vi "Settings Dialog.vi"(8 "error in (no error)":errorcluster, 11 "Settings in":T1={"Hardware Configuration"={"Sensor Channels"="", "Max Input"=10.0, "Min Input"=-10.0, "Sample Rate"=1000.0, "DAQmx Task"="", "Reference Channels"=""}, "Ga"=0.0, "Gv"=0.0, "ExportPath"=""}) -> (0 "error out":errorcluster, 1 "Cancelled?":bool=TRUE, 2 "UI Refresh Needed?":bool, 3 "Settings out":T1={"Hardware Configuration"={"Sensor Channels"="", "Max Input"=10.0, "Min Input"=-10.0, "Sample Rate"=1000.0, "DAQmx Task"="", "Reference Channels"=""}, "Ga"=0.0, "Gv"=0.0, "ExportPath"=""})   [LabVIEW 2017, in "Settings.lvlib"]
doc: "Dialog for selecting user specified settings."
uses:
  Settings.lvlib
  Settings.ctl
  Acquisition/Hardware Configuration.ctl
  <vilib>/Utility/xml.llb/Write to XML File(string).vi
  Acquisition/Acquisition.lvlib
panel:
  in  "Export Path":path
  in  "Reference G[V/m/s^2]":dbl=1000.0
  in  "Target G[V/m/s]":dbl=-10.0
  in  "Reference Channel":tag="Dev1/ai0"
  in  "Sample Rate":dbl=1000.0
  in  "Minimum Input":dbl=-10.0
  in  "Maximum Input":dbl=10.0
  in  "Sensor Channels":tag="Dev1/ai0"
  in  "Cancel Button":bool
  in  "OK Button":bool
  # "Non visible portion of dialog (needed for connector pane)."
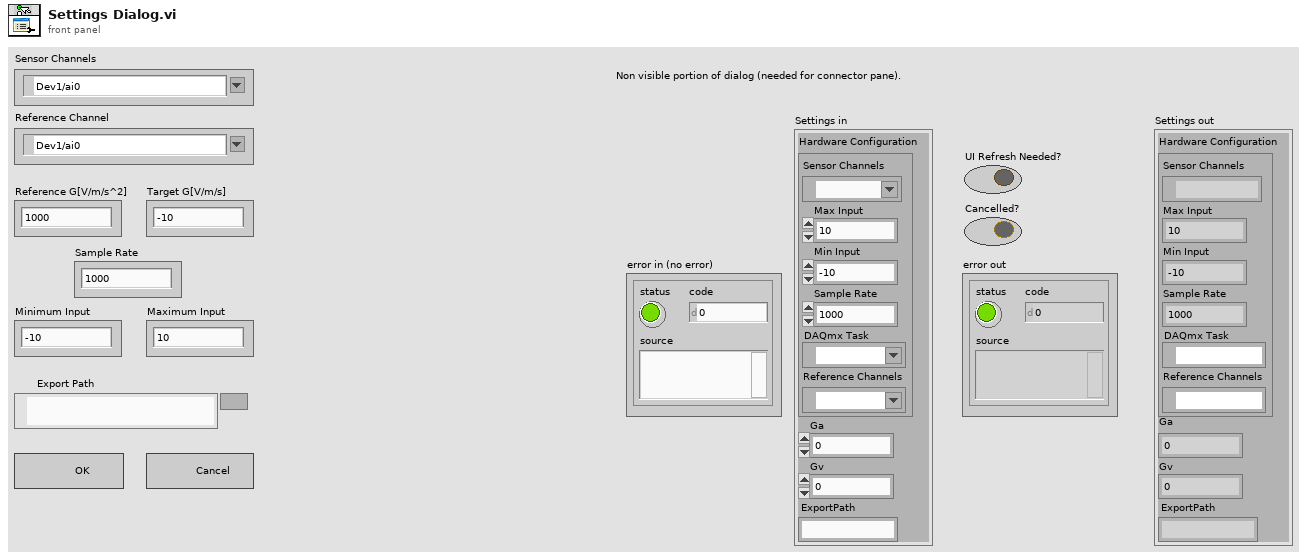
[diagram p1: front panel]
types:
  T1 = typedef "Settings.lvlib/Settings.ctl" = cluster{"Hardware Configuration":T2, "Ga":dbl, "Gv":dbl, "ExportPath":string}
  T2 = typedef "Acquisition.lvlib/Hardware Configuration.ctl" = cluster{"Sensor Channels":tag, "Max Input":dbl, "Min Input":dbl, "Sample Rate":dbl, "DAQmx Task":refnum<k21>, "Reference Channels":tag}
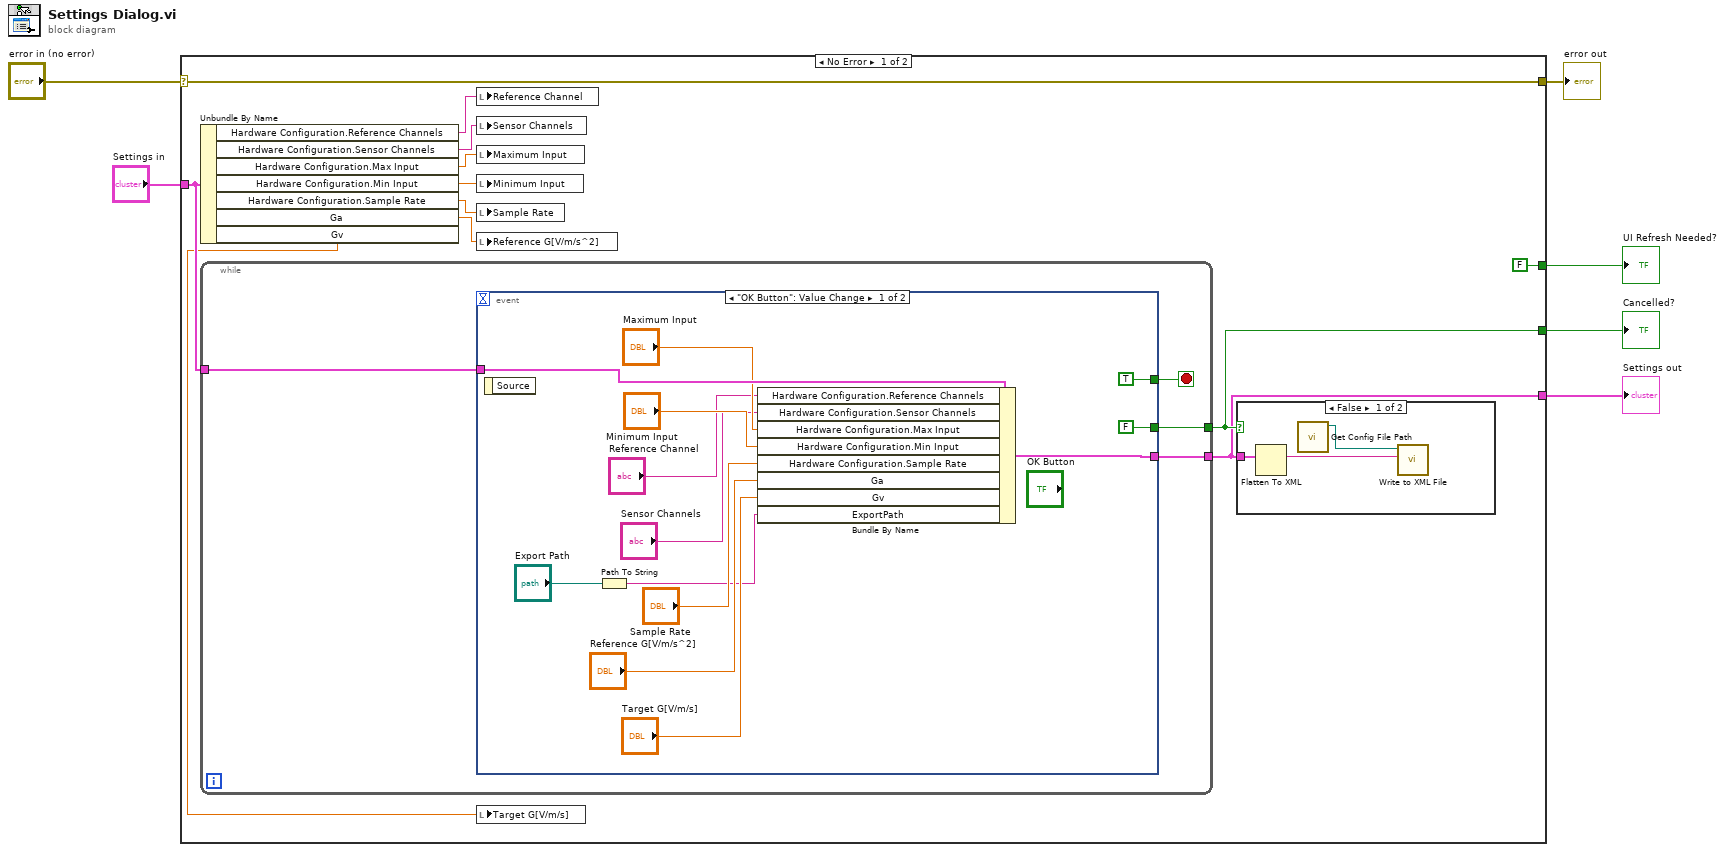
[diagram p0: block diagram]
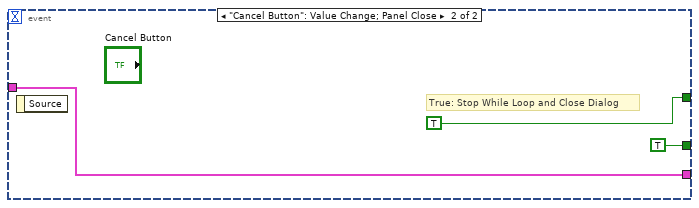
[diagram p2: hidden frame]
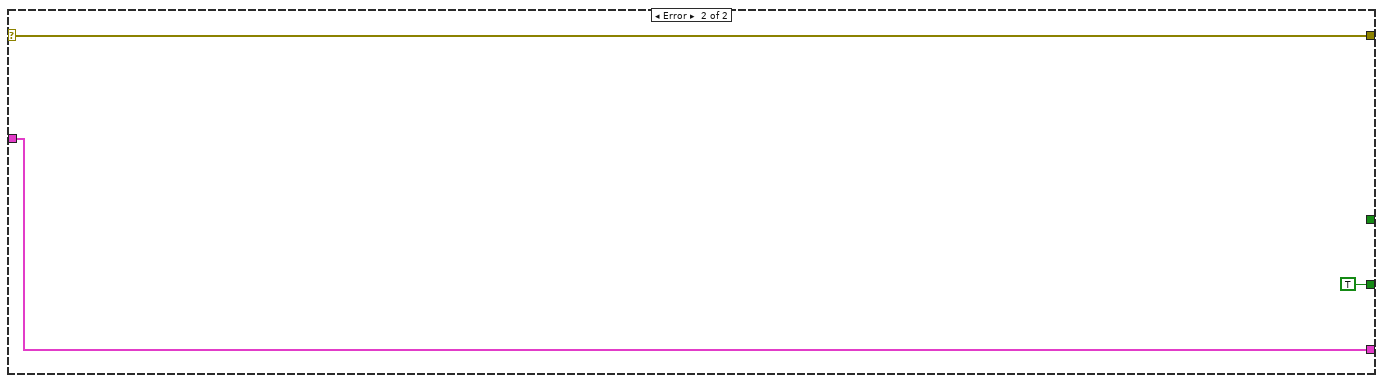
[diagram p4: hidden frame]
diagram:
  n1 = case shown="No Error" "error in (no error)" {
    selector: "error in (no error)" -> [w18 w44]
    tunnel: [w18 w44] -> w6
    tunnel: "Settings in" -> [w10 w43]
    tunnel: [w15 w43] -> w1
    tunnel: [FALSE ("UI Refresh Needed?") _] -> w4
    tunnel: [w16 TRUE ("UI Refresh Needed?")] -> w3
    frame No Error {
      n2 = Unbundle By Name(w10) -> ("Hardware Configuration.Reference Channels"=w9:tag, "Hardware Configuration.Sensor Channels"=w11:tag, "Hardware Configuration.Max Input"=w12:dbl, "Hardware Configuration.Min Input"=w13:dbl, "Hardware Configuration.Sample Rate"=w14:dbl, "Ga"=w8:dbl, "Gv"=w7:dbl)
      n3 = while {
        tunnel: [w22] -> w16
        tunnel: [w21] -> w15
        tunnel: w10 -> [w20]
        stop <- w19 stop-if-true
        n4 = event shown="[0] \"OK Button\": Value Change" {
          selector: _ -> [_ _]
          dyn-events: _ -> [_ _]
          timeout: _ -> [_ _]
          tunnel: [w33 w38] -> w21
          tunnel: w20 -> [w32 w38]
          tunnel: [FALSE ("UI Refresh Needed?") TRUE ("UI Refresh Needed?")] -> w22
          tunnel: [TRUE TRUE] -> w19
          event "OK Button": Value Change {
            n5 = event-data() -> ()  [unwired: 1 in, 1 out]
            n6 = Path To String(path="Export Path") -> (string=w23:string)
            n7 = Bundle By Name(cluster=w32, "Hardware Configuration.Reference Channels"="Reference Channel", "Hardware Configuration.Sensor Channels"="Sensor Channels", "Hardware Configuration.Max Input"="Maximum Input", "Hardware Configuration.Min Input"="Minimum Input", "Hardware Configuration.Sample Rate"="Sample Rate", "Ga"="Reference G[V/m/s^2]", "Gv"="Target G[V/m/s]", "ExportPath"=w23) -> (w33:T1)
          }
          event "Cancel Button": Value Change; Panel Close {
            # "True: Stop While Loop and Close Dialog"
            n8 = event-data() -> ()  [unwired: 1 in, 1 out]
          }
        }
      }
      n9 = local write "Reference Channel"(w9) -> ()
      n10 = local write "Sensor Channels"(w11) -> ()
      n11 = local write "Maximum Input"(w12) -> ()
      n12 = local write "Minimum Input"(w13) -> ()
      n13 = local write "Sample Rate"(w14) -> ()
      n14 = local write "Reference G[V/m/s^2]"(w8) -> ()
      n15 = local write "Target G[V/m/s]"(w7) -> ()
      n16 = case shown="False" w16 {
        tunnel: w15 -> [w40 _]
        frame False {
          n17 = Flatten To XML(anything=w40) -> (xml string=w39:string)
          n18 = call "Get Config File Path.vi"() -> ("XML File Path"=w41:path)  [unwired: 10 in, 1 out]
          n19 = call-poly <vilib>:"Write to XML File.vi"("XML Input"=w39, "XML File Path"=w41) -> ()  [unwired: 7 in, 3 out]
        }
        frame True {
        }
      }
    }
    frame Error {
    }
  }
  "UI Refresh Needed?" <- w4
  "error out" <- w6
  "Settings out" <- w1
  "Cancelled?" <- w3
